vi "SLL DE Create Directories.vi"(8 "error in (no error)":errorcluster, 11 "Filepath In":path) -> (0 "error out":errorcluster, 2 "Parent Directories":path[](array[path]), 3 "Dup File Path Out":path)   [LabVIEW 2013]
doc: "This VI gets the directory path and checks if the root directory is a valid.When it is valid it checks if the given directory's in the path exists.If the directory's does not exist it creates a new one. It also generates an array of all parent directories"
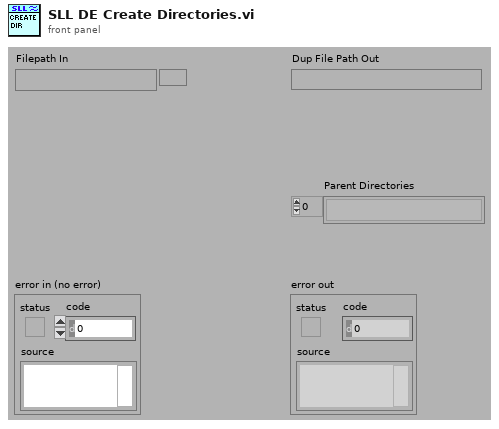
[diagram p1: front panel]
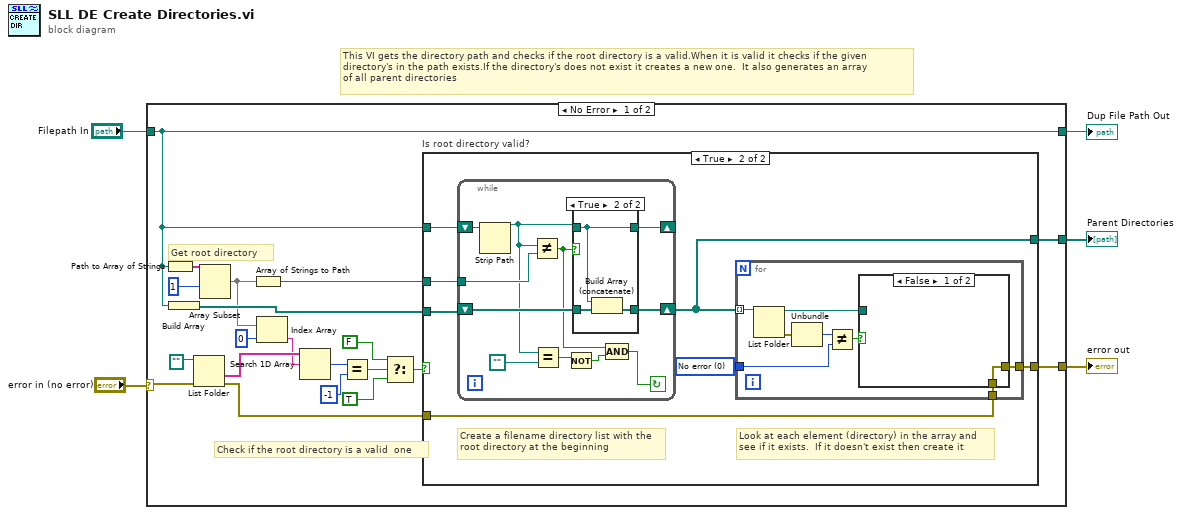
[diagram p0: block diagram]
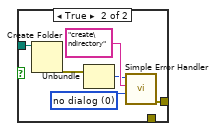
[diagram p4: hidden frame]
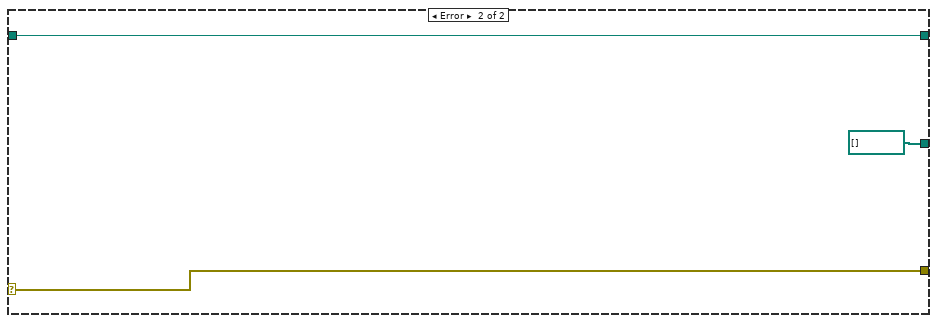
[diagram p5: hidden frame]
diagram:
  # "This VI gets the directory path and checks if the root directory is a valid.When it is valid it checks if the given \ndirectory's in the path exists.If the directory's does not exist it creates a new one.  It also generates an array \nof all parent directories"
  n1 = case shown="No Error" "error in (no error)" {
    selector: "error in (no error)" -> [w17 w65]
    tunnel: [w24 path[] []] -> w5
    tunnel: "Filepath In" -> [w20 w67]
    tunnel: [w20 w67] -> w3
    tunnel: [w19 w65] -> w2
    frame No Error {
      # "Check if the root directory is a valid  one"
      # "Get root directory"
      n2 = Path to Array of Strings(0:w20) -> (2:w23:string[])  [unwired: 1 out]
      n3 = Build Array(w20) -> (w25:path[])
      n4 = List Folder(path=path "", error in=w17) -> (folder names=w15:string[], error out=w16:errorcluster)  [unwired: 2 in, 2 out]
      n5 = Array Subset(array=w23, length=1) -> (w8:string[])  [unwired: 1 in]
      n6 = Array of Strings to Path(0:w8) -> (2:w22:path)  [unwired: 1 in]
      n7 = Index Array(array=w8, index=0) -> (element=w6:string)
      n8 = Search 1D Array(1D array=w15, element=w6) -> (index of element=w14:i32)  [unwired: 1 in]
      n9 = Equal?(x=w14, y=-1) -> (x = y?=w12:bool)
      n10 = Select(t=FALSE, s=w12, f=TRUE) -> (s? t:f=w9:bool)
      n11 = case "Is root directory valid?" shown="True" w9 {
        tunnel: w25 -> [_ w33]
        tunnel: [_ w32] -> w24
        tunnel: w22 -> [_ w30]
        tunnel: w20 -> [_ w29]
        tunnel: [w26 w28] -> w19
        tunnel: w16 -> [w26 w27]
        frame False {
        }
        frame True {
          w31 = 0 items=["No error", "Argument error", "Memory is full", "Out of zone", "End of file", "File already open", "Generic file I/O error", "File not found", "File permission error", "Disk is full", "Duplicate path", "Too many files open", "System feature not enabled", "Resource file not found", "Cannot add resource", "Resource not found", "Image not found", "Image memory error", "Pen does not exist", "Config type invalid", "Config token not found", "Config parse error", "Config memory error", "Bad external code format", "Bad external code offset", "External code not present", "Null window", "Destroy window error", "Null menu", "Print aborted", "Bad print record", "Print driver error", "Windows error during printing", "Memory error during printing", "Print dialog error", "Generic print error", "Invalid device refnum", "Device not found", "Device parameter error", "Device unit error", "Cannot open device", "Device call aborted", "Generic error", "Cancelled by user", "Object ID too low", "Object ID too high", "Object not in heap", "Unknown heap", "Unknown object (invalid DefProc)", "Unknown object (DefProc not in table)", "Message out of range", "Invalid (null) method", "Unknown message", "Manager call not supported", "Bad address", "Connection in progress", "Connection timed out", "Connection is already in progress", "Network attribute not supported", "Network error", "Address in use", "System out of memory", "Connection aborted", "Connection refused", "Not connected", "Already connected", "Connection closed", "Initialization error (interapplication manager)", "Bad occurrence", "Wait on unbound occurrence handler", "Occurrence queue overflow", "Datalog type conflict", "Unused", "Unrecognized type (interapplication manager)", "Memory corrupt", "Failed to make temporary DLL", "Old CIN version", "Unknown error code"]
          # "Look at each element (directory) in the array and\nsee if it exists.  If it doesn't exist then create it"
          # "Create a filename directory list with the\nroot directory at the beginning"
          n12 = while {
            tunnel: w30 -> [w40]
            shift-left: w29 -> [w41]
            shift-right: [w42] -> _
            shift-left: w33 -> [w44]
            shift-right: [w43] -> w32
            stop <- w34 continue-if-true
            n13 = Strip Path(path=w41) -> (stripped path=w39:path)  [unwired: 1 out]
            n14 = Not Equal?(x=w39, y=w40) -> (x != y?=w37:bool)
            n15 = Equal?(x=w39, y=path "") -> (x = y?=w36:bool)
            n16 = Not(x=w36) -> (.not. x?=w35:bool)
            n17 = case shown="True" w37 {
              tunnel: w44 -> [w46 w48]
              tunnel: [w46 w49] -> w43
              tunnel: w39 -> [w45 w47]
              tunnel: [w45 w47] -> w42
              frame False {
              }
              frame True {
                n18 = Build Array (concatenate)(w47, w48) -> (w49:path[])
              }
            }
            n19 = Compound Arithmetic op=AND(w37, w35) -> (w34:bool)
          }
          n20 = for {
            tunnel: w32 -> [w57] mode=indexing
            tunnel: w31 -> [w53]
            tunnel: [w51] -> w28
            tunnel: w27 -> [w50]
            n21 = List Folder(path=w57) -> (path out=w54:path, error out=w56:errorcluster)  [unwired: 3 in, 2 out]
            n22 = Unbundle(w56) -> ("code"=w52:i32)  [unwired: 2 out]
            n23 = Not Equal?(x=w52, y=w53) -> (x != y?=w55:bool)
            n24 = case shown="False" w55 {
              tunnel: w54 -> [_ w64]
              tunnel: [w58 w59] -> w51
              tunnel: w50 -> [w58 _]
              frame False {
              }
              frame True {
                w60 = u16 0 items=["no dialog", "OK message", "continue or stop message"] ("type of dialog (OK msg:1)")
                n25 = Create Folder(path (use dialog)=w64) -> (error out=w63:errorcluster)  [unwired: 2 in, 2 out]
                n26 = Unbundle(w63) -> ("code"=w61:i32)  [unwired: 2 out]
                n27 = call <vilib>:"Simple Error Handler.vi"("error code (no error:0)"=w61, "error source (\" \")"="create\ndirectory", "type of dialog (OK msg:1)"=w60) -> ("error out"=w59:errorcluster)  [unwired: 2 in, 4 out]
              }
            }
          }
        }
      }
    }
    frame Error {
    }
  }
  "Parent Directories" <- w5
  "Dup File Path Out" <- w3
  "error out" <- w2
